vi "Initialize.vi"(0 "FM Sweep in":refnum<class "FM Sweep.lvclass">, 1 "Filter in":refnum<class "Filter.lvclass">, 5 "Level in":refnum<class "Level.lvclass">, 7 "Fs (Hz)":dbl, 9 "Npts":i32, 11 "error in (no error)":errorcluster, 13 "Channel Name":string) -> (3 "Filter out":refnum<class "Filter.lvclass">, 4 "FM Sweep out":refnum<class "FM Sweep.lvclass">, 6 "Level out":refnum<class "Level.lvclass">, 15 "error out":errorcluster)   [LabVIEW 2020, in "FM Sweep.lvclass"]
uses:
  FM Sweep.lvclass
  Level/Level.lvclass
  Filter/Filter.lvclass
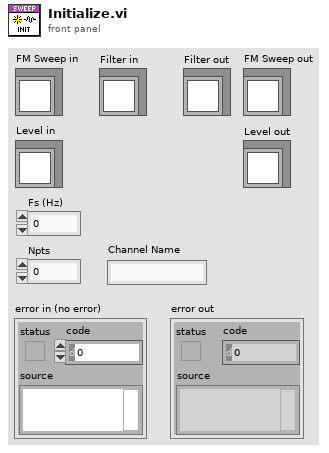
[diagram p1: front panel]
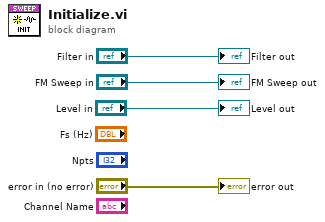
[diagram p0: block diagram]
diagram:
  "error out" <- "error in (no error)"
  "FM Sweep out" <- "FM Sweep in"
  "Level out" <- "Level in"
  "Filter out" <- "Filter in"
